vi "DVR.testMode.Read.vi"(6 "DVR in":T1) -> (1 "timeout":i32)   [LabVIEW 2020]
uses:
  _controls/data.ctl
  camera/camera.lvclass
  _controls/data.ref.ctl
  <vilib>/vision/Image Controls.llb/IMAQ Image.ctl
  _controls/state.ctl
  _controls/data.vars.ctl
  _controls/save_options.ctl
  _controls/flip.ctl
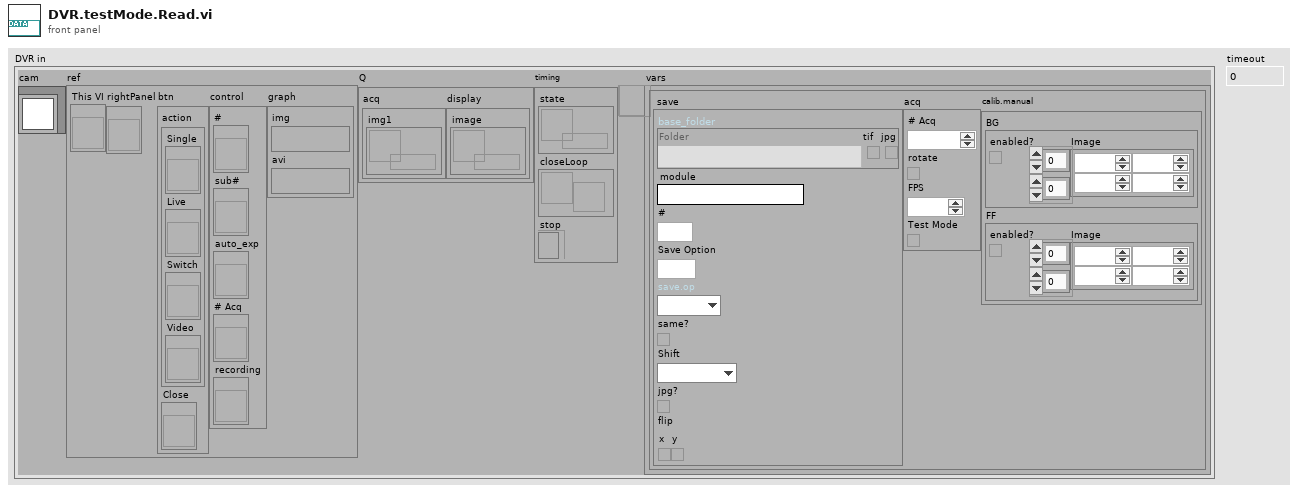
[diagram p1: front panel]
types:
  T1 = typedef "data.ctl" = cluster{"cam":refnum<class "camera.lvclass">, "ref":T2, "Q":cluster{"acq":cluster{"img1":refnum<queue>}, "display":cluster{"image":refnum<queue>}}, "timing":cluster{"state":refnum<queue>, "closeLoop":refnum<notifier>, "stop":refnum<k4>}, "vars":refnum<data-value>}
  T2 = typedef "data.ref.ctl" = cluster{"This VI":refnum<vi>, "rightPanel":refnum<vi>, "btn":cluster{"action":cluster{"Single":refnum<vi>, "Live":refnum<vi>, "Switch":refnum<vi>, "Video":refnum<vi>}, "Close":refnum<vi>}, "control":cluster{"#":refnum<vi>, "sub#":refnum<vi>, "auto_exp":refnum<vi>, "# Acq":refnum<vi>, "recording":refnum<vi>}, "graph":cluster{"img":T3, "avi":T3}}
  T3 = typedef "IMAQ Image.ctl" = refnum<image>
  T4 = typedef "data.vars.ctl" = cluster{"save":cluster{"base_folder":cluster{"Folder":path, "tif":bool, "jpg":bool}, "module":string, "#":u32, "sub#":u8, "save.op":T5, "same?":bool, "Shift":enum16{"Single", "Leapfrog"}, "jpg?":bool, "flip":T6}, "acq":cluster{"# Acq":u16, "rotate":bool, "FPS":dbl, "Test Mode":bool}, "calib.manual":cluster{"BG":cluster{"Image":u16[][], "enabled?":bool}, "FF":cluster{"Image":u16[][], "enabled?":bool}}}
  T5 = typedef "save_options.ctl" = enum16{"Light", "Full"}
  T6 = typedef "flip.ctl" = cluster{"x":bool, "y":bool}
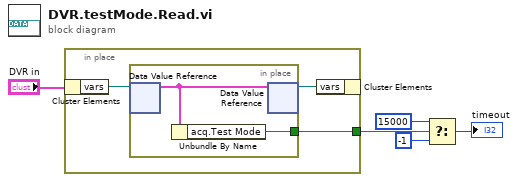
[diagram p0: block diagram]
diagram:
  n1 = in-place {
    in-place-border: [w6] -> w4
    n2 = in-place-cluster #1("DVR in") -> ("vars"=w8:refnum<data-value>)
    n3 = in-place {
      in-place-border: [w9] -> w6
      n4 = in-place-dvr #2(w8) -> (w10:T4)  [unwired: 1 out]
      n5 = Unbundle By Name(w10) -> ("acq.Test Mode"=w9:bool)
      n6 = in-place-dvr #2(w10) -> (w7:refnum<data-value>)  [unwired: 1 out]
    }
    n7 = in-place-cluster #1("vars"=w7) -> ()  [unwired: 1 out]
  }
  n8 = Select(t=15000, s=w4, f=-1) -> (s? t:f=→"timeout":i32)
